vi "HeaterWrite.vi"(8 "Error In":errorcluster, 11 "Omega CSi32 In":refnum<visa-resource-name>) -> (0 "Error Out":errorcluster, 3 "Omega CSi32 Out":refnum<visa-resource-name>)   [LabVIEW 2012]
uses:
  HeaterConfigurationGlobalAction.ctl
  libs/Omega-CSi32/Omega-CSi32.lvlib
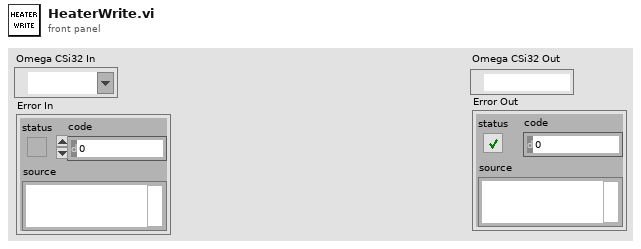
[diagram p1: front panel]
types:
  T1 = typedef "HeaterConfigurationGlobalAction.ctl" = enum16{"Init", "Get", "Set", "Add", "Remove", "Reset"}
  T2 = typedef "HeaterConfiguration.ctl" = cluster{"VISA Resource":refnum<visa-resource-name>, "COM Port":u8, "Setpoint":dbl, "Standby?":bool}
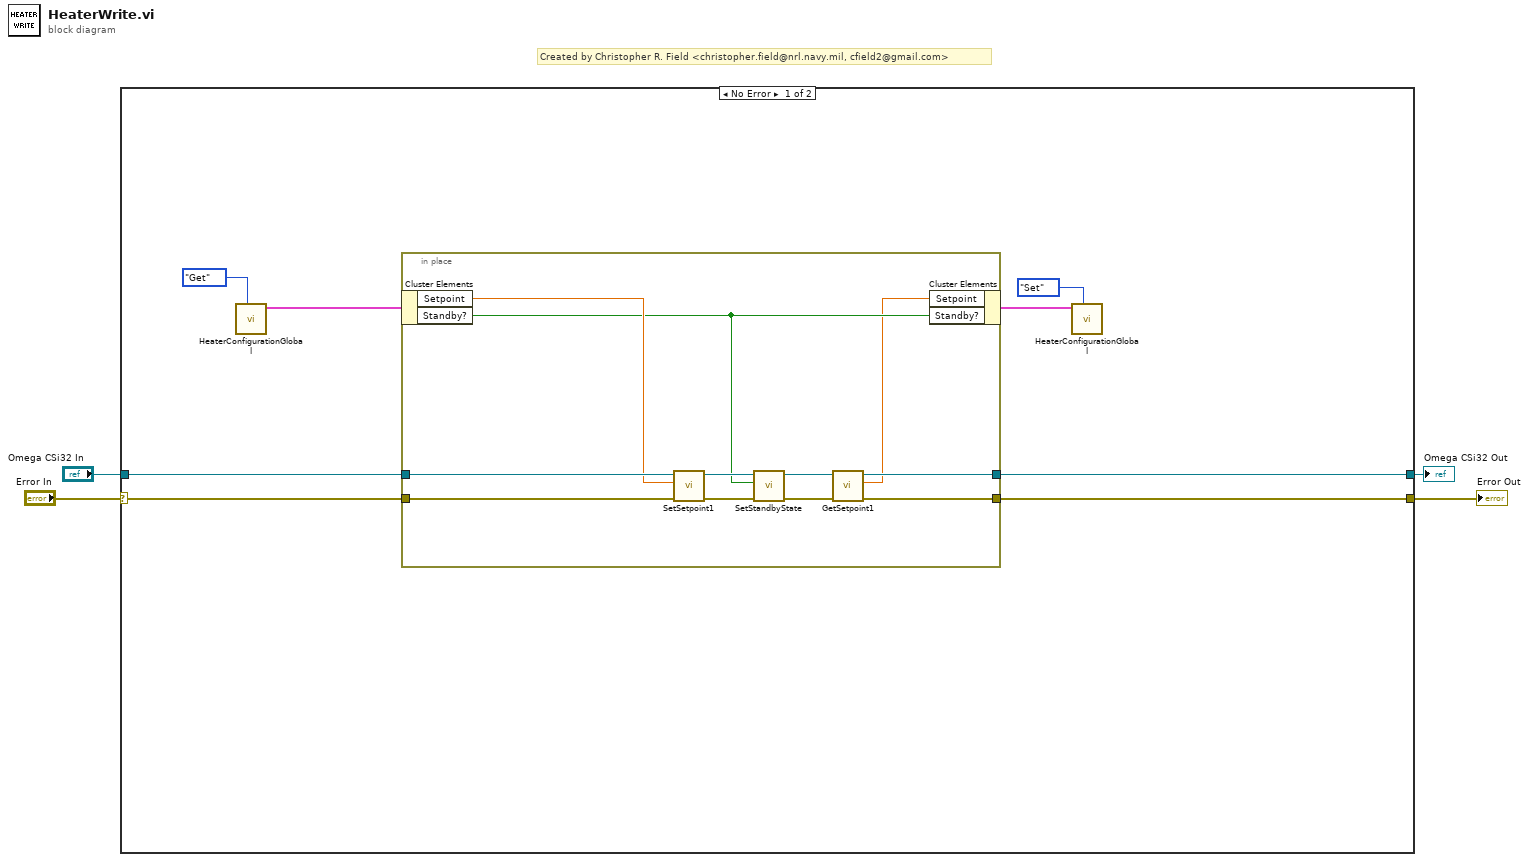
[diagram p0: block diagram]
diagram:
  # "Created by Christopher R. Field <christopher.field@nrl.navy.mil, cfield2@gmail.com>"
  n1 = case shown="No Error" "Error In" {
    selector: "Error In" -> [w12 w24]
    tunnel: "Omega CSi32 In" -> [w11 w25]
    tunnel: [w8 w25] -> w2
    tunnel: [w7 w24] -> w1
    frame No Error {
      n2 = call "HeaterConfigurationGlobal.vi"("Action"=HeaterConfigurationGlobalAction."Get") -> ("Value Out"=w6:T2)  [unwired: 8 in, 2 out]
      n3 = in-place {
        in-place-border: w12 -> [w19]
        in-place-border: w11 -> [w18]
        in-place-border: [w17] -> w8
        in-place-border: [w16] -> w7
        n4 = in-place-cluster #1(w6) -> ("Setpoint"=w15:dbl, "Standby?"=w14:bool)
        n5 = call "SetSetpoint1.vi"("Error In"=w19, "Setpoint (C)"=w15, "Omega CSi32 In"=w18) -> ("Error Out"=w21:errorcluster, "Omega CSi32 Out"=w20:refnum<visa-resource-name>)  [unwired: 7 in]
        n6 = call "SetStandbyState.vi"("Error In"=w21, "Enable"=w14, "Omega CSi32 In"=w20) -> ("Error Out"=w22:errorcluster, "Omega CSi32 Out"=w23:refnum<visa-resource-name>)  [unwired: 7 in]
        n7 = call "GetSetpoint1.vi"("Error In"=w22, "Omega CSi32 In"=w23) -> ("Error Out"=w16:errorcluster, "Setpoint 1 (C)"=w13:dbl, "Omega CSi32 Out"=w17:refnum<visa-resource-name>)  [unwired: 7 in]
        n8 = in-place-cluster #1("Setpoint"=w13, "Standby?"=w14) -> (w5:T2)
      }
      n9 = call "HeaterConfigurationGlobal.vi"("Action"=HeaterConfigurationGlobalAction."Set", "Set Value"=w5) -> ()  [unwired: 7 in, 3 out]
    }
    frame Error {
    }
  }
  "Omega CSi32 Out" <- w2
  "Error Out" <- w1
